vi "dequeueEncoder.vi"(8 "error in (no error)":errorcluster) -> (0 "error out":errorcluster, 3 "String":string)   [LabVIEW 2017, in "externalAquisition.lvlib"]
uses:
  externalAquisition.lvlib
  TypeDefs/QueueCommands.ctl
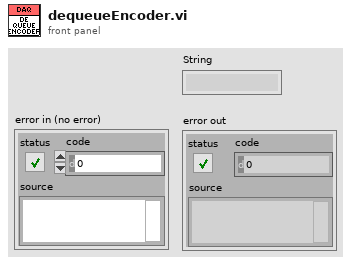
[diagram p1: front panel]
types:
  T1 = typedef "externalAquisition.lvlib/QueueCommands.ctl" = enum16{"get", "set"}
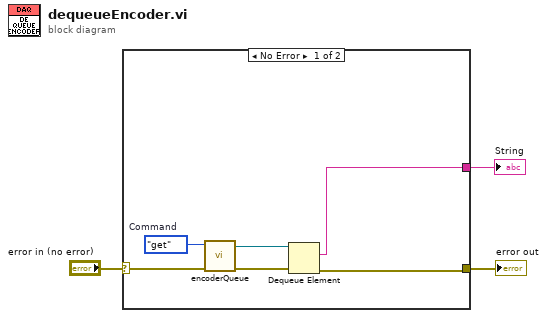
[diagram p0: block diagram]
diagram:
  n1 = case shown="No Error" "error in (no error)" {
    selector: "error in (no error)" -> [w9 w10]
    tunnel: [w5 w10] -> w2
    tunnel: [w4 _] -> w1
    frame No Error {
      w8 = QueueCommands."get"  # Command
      n2 = call "encoderQueue.vi"("error in (no error)"=w9, "Command"=w8) -> ("error out"=w6:errorcluster, "queue out"=w7:refnum<queue>)  [unwired: 8 in]
      n3 = Dequeue Element(queue=w7, error in (no error)=w6) -> (element=w4:string, error out=w5:errorcluster)  [unwired: 1 in, 2 out]
    }
    frame Error {
    }
  }
  "error out" <- w2
  "String" <- w1
